vi "FB Switch Input Var Read.vi"(8 "error in":errorcluster) -> (0 "error out":errorcluster, 3 "data out":variant)   [LabVIEW 2017]
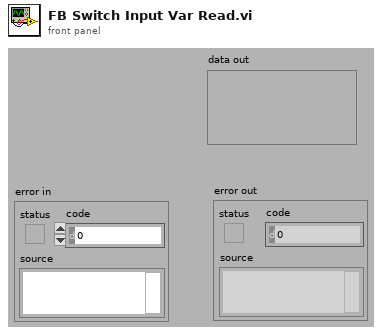
[diagram p1: front panel]
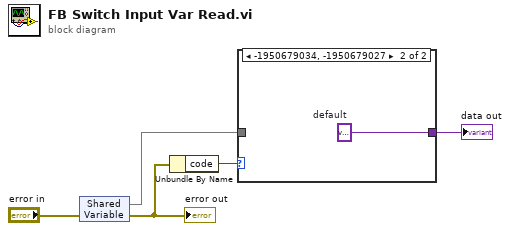
[diagram p0: block diagram]
diagram:
  n1 = shared-variable(error in="error in") -> (w1, error out=w4:errorcluster)
  "error out" <- w4
  n2 = Unbundle By Name(w4) -> ("code"=w3:i32)
  n3 = case shown="-1950679034, -1950679027" w3 {
    tunnel: w1 -> [w6 _]
    tunnel: [w6 w7] -> w2
    frame Default {
    }
    frame -1950679034, -1950679027 {
      w7 = variant  # default
    }
  }
  "data out" <- w2
